vi "Part 1.vi"(11 "Input":string) -> (3 "Output":i64)   [LabVIEW 2021]
uses:
  4da5fc84-eb69-4437-9412-81deace973a0.vi
  <userlib>/_OpenG.lib/string/string.llb/Convert EOLs (String)__ogtk.vi
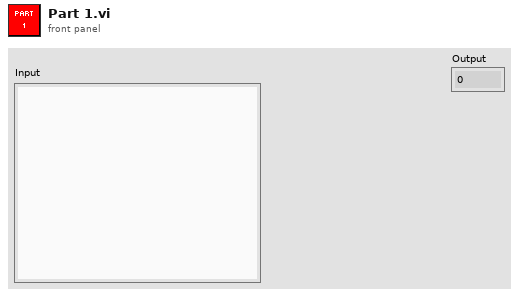
[diagram p1: front panel]
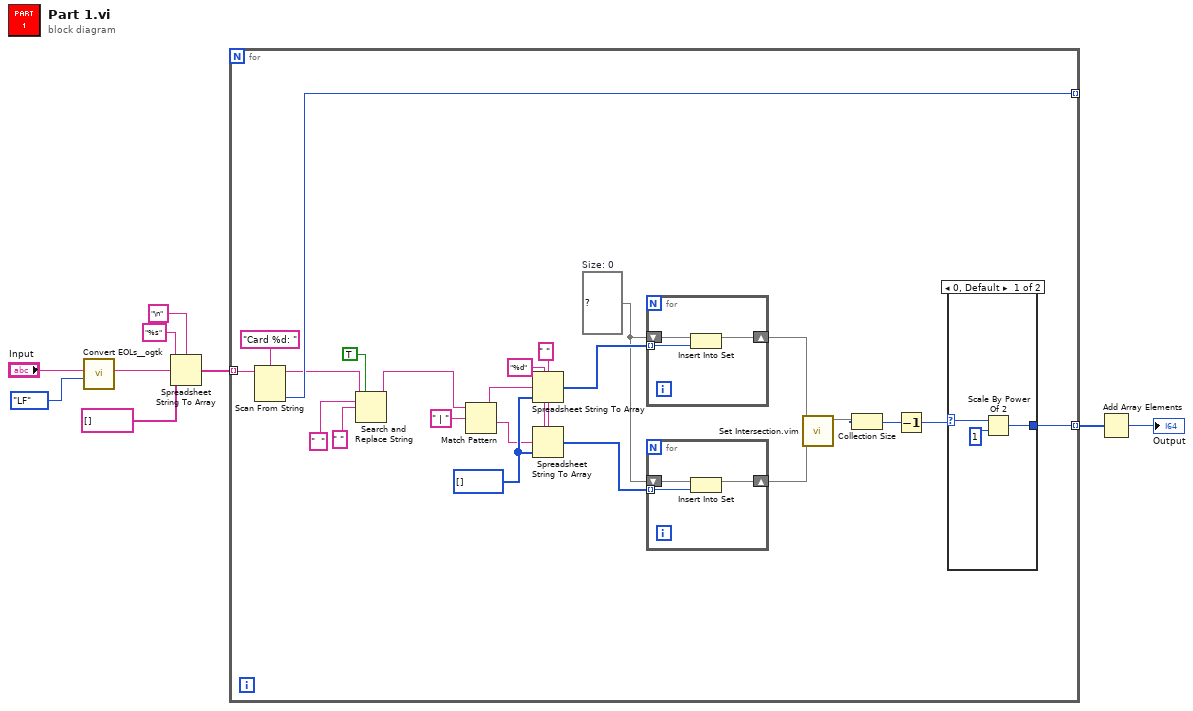
[diagram p0: block diagram]
diagram:
  n1 = call-poly <userlib>:"Convert EOLs__ogtk.vi"("Convert to:"=enum16{"CR", "LF", "CRLF"}."LF", "String in"="Input") -> ("String out"=w5:string)  [unwired: 9 in]
  n2 = Spreadsheet String To Array(delimiter (Tab)="\n", format string="%s", spreadsheet string=w5, array type (2D Dbl)=string[] []) -> (array=w3:string[])
  n3 = for {
    tunnel: w3 -> [w32] mode=indexing
    tunnel: [w30] -> _ mode=indexing
    tunnel: [w10] -> w2 mode=indexing
    w17 = set{i64} {}  # Size: 0
    w24 = " "
    w25 = "%d"
    w28 = i64[] []
    n4 = Scan From String(format string="Card %d: ", input string=w32) -> (remaining string=w23:string, output 1=w30:i32)  [unwired: 3 in, 2 out]
    n5 = Search and Replace String(replace all?=TRUE, input string=w23, search string="  ", replace string=" ") -> (result string=w22:string)  [unwired: 4 in, 3 out]
    n6 = Match Pattern(string=w22, regular expression=" | ") -> (before substring=w26:string, after substring=w27:string)  [unwired: 1 in, 2 out]
    n7 = Spreadsheet String To Array(delimiter (Tab)=w24, format string=w25, spreadsheet string=w26, array type (2D Dbl)=w28) -> (array=w18:i64[])
    n8 = Spreadsheet String To Array(delimiter (Tab)=w24, format string=w25, spreadsheet string=w27, array type (2D Dbl)=w28) -> (array=w16:i64[])
    n9 = for {
      tunnel: w18 -> [w41] mode=indexing
      shift-right: [w40] -> w14
      shift-left: w17 -> [w39]
      n10 = Insert Into Set(10:w41, 11:w39) -> (3:w40:set{i64})  [unwired: 1 out]
    }
    n11 = for {
      tunnel: w16 -> [w38] mode=indexing
      shift-right: [w37] -> w15
      shift-left: w17 -> [w36]
      n12 = Insert Into Set(10:w38, 11:w36) -> (3:w37:set{i64})  [unwired: 1 out]
    }
    n13 = call "Set Intersection.vim"("set 2"=w15, "set 1"=w14) -> ("intersection"=w13:set{i64})  [unwired: 9 in]
    n14 = Collection Size(1:w13) -> (0:w12:i32)
    n15 = Decrement(x=w12) -> (x-1=w11:i32)
    n16 = case shown="0, Default" w11 {
      selector: w11 -> [w35 _]
      tunnel: [w33 _] -> w10
      frame 0, Default {
        n17 = Scale By Power Of 2(n=w35, x=i64 1) -> (x*2^n=w33:i64)
      }
      frame -1 {
      }
    }
  }
  n18 = Add Array Elements(numeric array=w2) -> (sum=→"Output":i64)
